vi "Close.vi"(8 "error in (no error)":errorcluster, 11 "dotNET SSL Socket in":refnum<class "dotNET SSL Socket.lvclass">) -> (0 "error out":errorcluster)   [LabVIEW 2013, in "dotNET SSL Socket.lvlib" / "dotNET SSL Socket.lvclass"]
doc: "Closes the socket connection.\nWebSockets 2.0.0.30\nSam Sharp - MediaMongrels Ltd\nCopyright (c) 2019, MediaMongrels Ltd"
uses:
  dotNET SSL Socket.lvclass
  dotNET SSL Socket.lvclass/dotNET SSL Socket.ctl
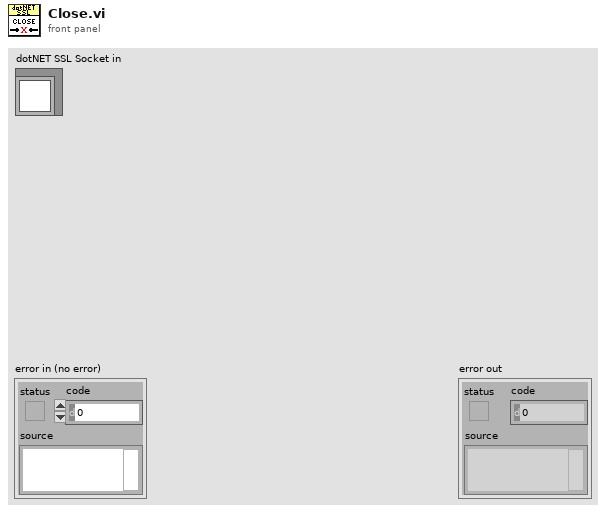
[diagram p1: front panel]
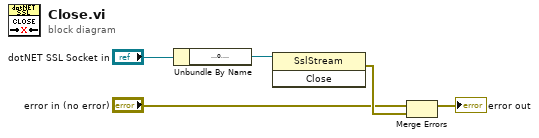
[diagram p0: block diagram]
diagram:
  n1 = Unbundle By Name("dotNET SSL Socket in") -> ("SSLStream"=w4:refnum<k24>)
  n2 = invoke class="SslStream" method="Close"(reference=w4) -> (error out=w3:errorcluster)  [unwired: 2 in, 2 out]
  n3 = Merge Errors("error in (no error)", w3) -> (→"error out":errorcluster)
